vi "Periodic Tasks.vi"(8 "error in":errorcluster) -> ()   [LabVIEW 2013]
doc: "This VI runs in parallel to other tasks. It can contain as many user-defined periodic loops as you need. These can carry out PID or other sorts of timed response."
uses:
  <vilib>/Rock Robotics/SystemInterfaces/Utilities/FPGA_UtilitiesLED Source.ctl
  <vilib>/Rock Robotics/SystemInterfaces/Utilities/FPGA_UtilitiesLED State.ctl
  Robot Global Data.vi
panel:
  out "Numeric":dbl
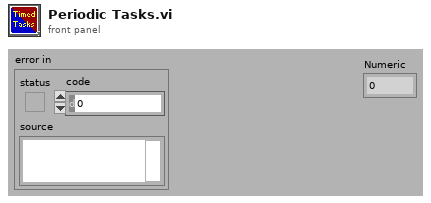
[diagram p1: front panel]
types:
  T1 = typedef "WPI_MotorControlDeviceRef.ctl" = cluster{"DeviceStatus":errorcluster, "Type":enum16{"PWM", "CAN"}, "PWM":cluster{"Digital Module":T2, "PWM Channel":T3, "DeadBand":T4}, "CAN":cluster{"Device Number":u8, "Control Mode":T5, "Semaphore":T6, "Max Vout":dbl}, "Invert":bool, "TransformRef":T7, "InvTransformRef":T7}
  T2 = typedef "FPGA_TypedefDigitalModule.ctl" = enum16{"Digital Module 1", "Digital Module 2"}
  T3 = typedef "FPGA_DIOPWMChannel.ctl" = enum8{"PWM 1", "PWM 2", "PWM 3", "PWM 4", "PWM 5", "PWM 6", "PWM 7", "PWM 8", "PWM 9", "PWM 10", "Invalid"}
  T4 = typedef "WPI_PWMDeadband.ctl" = cluster{"Name":string, "maxPositivePwm":i32, "minPositivePwm":i32, "centerPwm":i32, "maxNegativePwm":i32, "minNegativePwm":i32, "angularRange":u16}
  T5 = typedef "WPI_CANJaguar_ControlMode.ctl" = enum8{"Percent VBus", "Current", "Speed", "Position", "Voltage"}
  T6 = typedef "Semaphore RefNum" = refnum<k1>
  T7 = typedef "WPI_PWMTransform_ConPane.ctl" = refnum<vi>
  T8 = typedef "FPGA_UtilitiesLED State.ctl" = enum16{"Off", "On", "Toggle"}
  T9 = typedef "FPGA_UtilitiesLED Source.ctl" = enum16{"User LED", "FPGA LED"}
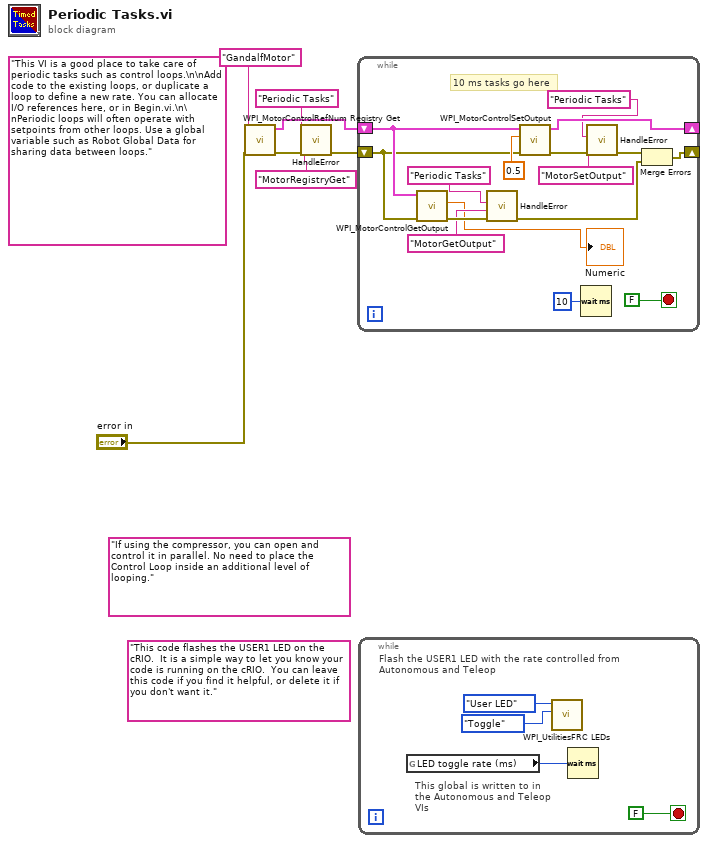
[diagram p0: block diagram]
diagram:
  (unwired) "If using the compressor, you can open and control it in parallel. No need to place the Control Loop inside an additional level of looping."
  (unwired) "This code flashes the USER1 LED on the cRIO.  It is a simple way to let you know your code is running on the cRIO.  You can leave this code if you find it helpful, or delete it if you don't want it."
  (unwired) "This VI is a good place to take care of periodic tasks such as control loops.\n\nAdd code to the existing loops, or duplicate a loop to define a new rate. You can allocate I/O references here, or in Begin.vi.\n\nPeriodic loops will often operate with setpoints from other loops. Use a global variable such as Robot Global Data for sharing data between loops."
  n1 = call <vilib>:"WPI_MotorControlRefNum Registry Get.vi"("error in (no error)"="error in", "refnum name"="GandalfMotor") -> ("error out"=w3:errorcluster, "MotorControlDevRef"=w6:T1)  [unwired: 8 in]
  n2 = call "HandleError.vi"("error in (no error)"=w3, "Causing VI"="MotorRegistryGet", "Calling VI"="Periodic Tasks") -> ("error out"=w4:errorcluster)  [unwired: 8 in]
  n3 = while {
    shift-right: [w20] -> _
    shift-left: w6 -> [w16]
    shift-right: [w13] -> _
    shift-left: w4 -> [w15]
    stop <- FALSE stop-if-true
    # "10 ms tasks go here"
    n4 = call <vilib>:"WPI_MotorControlGetOutput.vi"("error in (no error)"=w15, "MotorControlDevRef"=w16) -> ("error out"=w12:errorcluster, "Output"=→"Numeric":dbl)  [unwired: 7 in, 1 out]
    n5 = call "HandleError.vi"("error in (no error)"=w12, "Causing VI"="MotorGetOutput", "Calling VI"="Periodic Tasks") -> ("error out"=w11:errorcluster)  [unwired: 8 in]
    n6 = call <vilib>:"WPI_MotorControlSetOutput.vi"("error in (no error)"=w15, "Output"=0.5, "MotorControlDevRef"=w16) -> ("error out"=w21:errorcluster, "MotorControlDevRef"=w20:T1)  [unwired: 6 in, 1 out]
    n7 = Wait (ms)(milliseconds to wait=u32 10) -> ()  [unwired: 1 out]
    n8 = call "HandleError.vi"("error in (no error)"=w21, "Causing VI"="MotorSetOutput", "Calling VI"="Periodic Tasks") -> ("error out"=w14:errorcluster)  [unwired: 8 in]
    n9 = Merge Errors(w14, w11) -> (w13:errorcluster)
  }
  n10 = while {
    stop <- FALSE stop-if-true
    # "This global is written to in the Autonomous and Teleop VIs"
    # "Flash the USER1 LED with the rate controlled from Autonomous and Teleop"
    n11 = global read "Robot Global Data.vi" "LED toggle rate (ms)"() -> (w24:u32)
    n12 = call <vilib>:"WPI_UtilitiesFRC LEDs.vi"("State"=FPGA_UtilitiesLED_State."Toggle", "LED Type"=FPGA_UtilitiesLED_Source."User LED") -> ()  [unwired: 1 in, 9 out]
    n13 = Wait (ms)(milliseconds to wait=w24) -> ()  [unwired: 1 out]
  }
